vi "DSF.Engine.Plugin.Rx.Inline.Start.vi"(8 "error in (no error)":errorcluster, 11 "Plugin in":refnum<class "DSF.Engine.Plugin.lvclass">) -> (0 "error out":errorcluster, 3 "Plugin out":refnum<class "DSF.Engine.Plugin.lvclass">)   [LabVIEW 2017, in "DSF.Engine.lvlib" / "DSF.Engine.Plugin.lvclass"]
uses:
  DSF.Engine.Plugin.lvclass
  DSF.Engine.Plugin.lvclass/DSF.Engine.Plugin.ctl
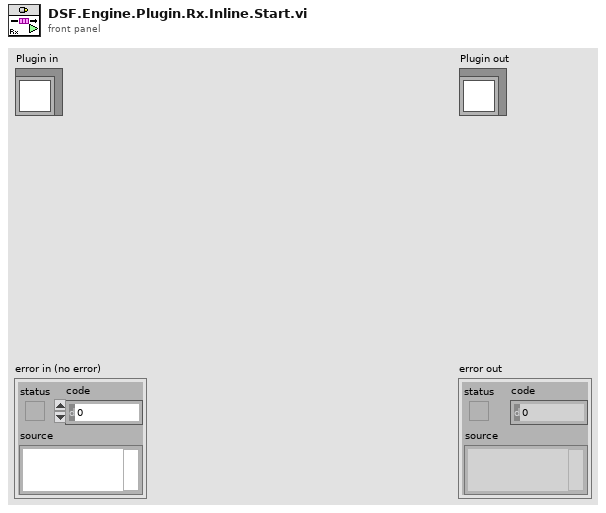
[diagram p1: front panel]
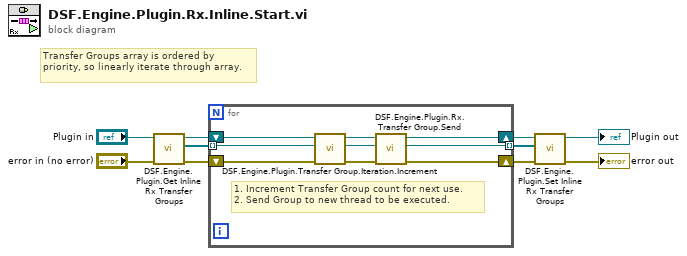
[diagram p0: block diagram]
diagram:
  # "Transfer Groups array is ordered by priority, so linearly iterate through array."
  n1 = call "DSF.Engine.Plugin.Get Inline Rx Transfer Groups.vi"("Plugin in"="Plugin in") -> ("Inline Rx Transfer Groups"=w8:refnum<class "DSF.Engine.Transfer Group.lvclass">[], "Plugin out"=w7:refnum<class "DSF.Engine.Plugin.lvclass">)  [unwired: 9 in]
  n2 = for {
    tunnel: w8 -> [w11] mode=indexing
    shift-right: [w16] -> w6
    shift-left: w7 -> [w10]
    shift-right: [w17] -> w2
    shift-left: "error in (no error)" -> [w9]
    tunnel: [w15] -> w5 mode=indexing
    # "1. Increment Transfer Group count for next use.\n2. Send Group to new thread to be executed."
    n3 = call "DSF.Engine.Plugin.Transfer Group.Iteration.Increment.vi"("error in (no error)"=w9, "Transfer Group in"=w11, "Plugin in"=w10) -> ("error out"=w13:errorcluster, "Transfer Group out"=w12:refnum<class "DSF.Engine.Transfer Group.lvclass">, "Plugin out"=w14:refnum<class "DSF.Engine.Plugin.lvclass">)  [unwired: 6 in]
    n4 = call "DSF.Engine.Plugin.Rx.Transfer Group.Send.vi"("error in (no error)"=w13, "Transfer Group in"=w12, "Plugin in"=w14) -> ("error out"=w17:errorcluster, "Transfer Group out"=w15:refnum<class "DSF.Engine.Transfer Group.lvclass">, "Plugin out"=w16:refnum<class "DSF.Engine.Plugin.lvclass">)  [unwired: 6 in]
  }
  "error out" <- w2
  n5 = call "DSF.Engine.Plugin.Set Inline Rx Transfer Groups.vi"("Inline Rx Transfer Groups"=w5, "Plugin in"=w6) -> ("Plugin out"=→"Plugin out":refnum<class "DSF.Engine.Plugin.lvclass">)  [unwired: 9 in]
